vi "BNC555.ProcEvents.vi"(0 "i ref in":refnum<vi>, 5 "error in":errorcluster) -> (14 "i ref out":refnum<vi>, 19 "error out":errorcluster)   [LabVIEW 2014, in "BNC555.lvlib"]
doc: "This method is used to define the events the object will listen to. Add your own events here."
uses:
  BNC555.lvlib
  CS_Core/BaseProcess/BaseProcess.event definition.ctl
  CS_Core/CAEObj/CAEObj.event definition.ctl
  CS_Core/BaseProcess/BaseProcess.descriptor string definition.ctl
  CS_Core/BaseProcess/BaseProcess.lvlib
  CS_Core/CAEObj/CAEObj.lvlib
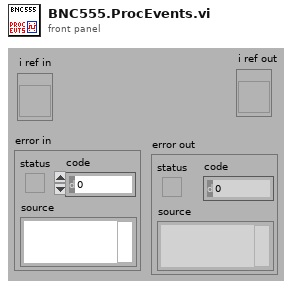
[diagram p1: front panel]
types:
  T1 = typedef "BaseProcess.lvlib/BaseProcess.event definition.ctl" = cluster{"CAEEvtDef":T2, "Data Descriptor":T3}
  T2 = typedef "CAEObj.lvlib/CAEObj.event definition.ctl" = cluster{"URL":string, "enable":bool, "ignoreResID":bool}
  T3 = typedef "BaseProcess.lvlib/BaseProcess.descriptor string definition.ctl" = string
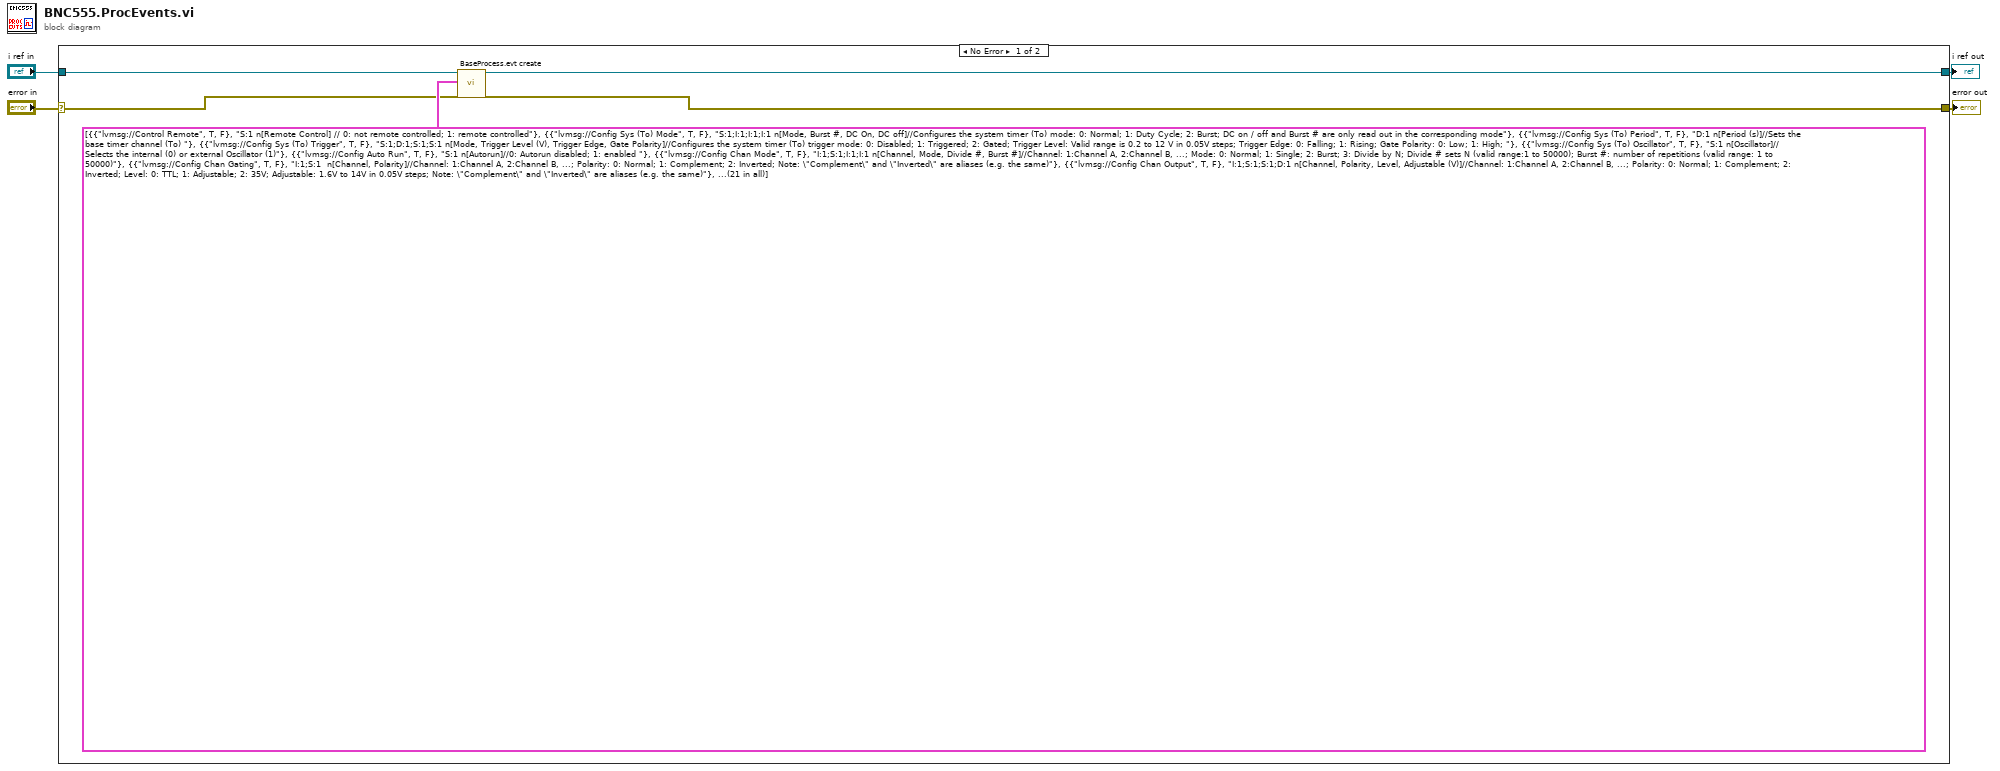
[diagram p0: block diagram]
diagram:
  n1 = case shown="No Error" "error in" {
    selector: "error in" -> [w5 w10]
    tunnel: "i ref in" -> [w9 w11]
    tunnel: [w8 w11] -> w3
    tunnel: [w7 w10] -> w2
    frame No Error {
      n2 = call "BaseProcess.evt create.vi"("i ref in"=w9, "newEvents"=T1[] [{"CAEEvtDef"={"URL"="lvmsg://Control Remote", "enable"=TRUE, "ignoreResID"=FALSE}, "Data Descriptor"="S:1 n[Remote Control] // 0: not remote controlled; 1: remote controlled"}, {"CAEEvtDef"={"URL"="lvmsg://Config Sys (To) Mode", "enable"=TRUE, "ignoreResID"=FALSE}, "Data Descriptor"="S:1;I:1;I:1;I:1 n[Mode, Burst #, DC On, DC off]//Configures the system timer (To) mode: 0: Normal; 1: Duty Cycle; 2: Burst; DC on / off and Burst # are only read out in the corresponding mode"}, {"CAEEvtDef"={"URL"="lvmsg://Config Sys (To) Period", "enable"=TRUE, "ignoreResID"=FALSE}, "Data Descriptor"="D:1 n[Period (s)]//Sets the base timer channel (To) "}, {"CAEEvtDef"={"URL"="lvmsg://Config Sys (To) Trigger", "enable"=TRUE, "ignoreResID"=FALSE}, "Data Descriptor"="S:1;D:1;S:1;S:1 n[Mode, Trigger Level (V), Trigger Edge, Gate Polarity]//Configures the system timer (To) trigger mode: 0: Disabled; 1: Triggered; 2: Gated; Trigger Level: Valid range is 0.2 to 12 V in 0.05V steps; Trigger Edge: 0: Falling; 1: Rising; Gate Polarity: 0: Low; 1: High; "}, {"CAEEvtDef"={"URL"="lvmsg://Config Sys (To) Oscillator", "enable"=TRUE, "ignoreResID"=FALSE}, "Data Descriptor"="S:1 n[Oscillator]//Selects the internal (0) or external Oscillator (1)"}, {"CAEEvtDef"={"URL"="lvmsg://Config Auto Run", "enable"=TRUE, "ignoreResID"=FALSE}, "Data Descriptor"="S:1 n[Autorun]//0: Autorun disabled; 1: enabled "}, {"CAEEvtDef"={"URL"="lvmsg://Config Chan Mode", "enable"=TRUE, "ignoreResID"=FALSE}, "Data Descriptor"="I:1;S:1;I:1;I:1 n[Channel, Mode, Divide #, Burst #]//Channel: 1:Channel A, 2:Channel B, ...; Mode: 0: Normal; 1: Single; 2: Burst; 3: Divide by N; Divide # sets N (valid range:1 to 50000); Burst #: number of repetitions (valid range: 1 to 50000)"}, {"CAEEvtDef"={"URL"="lvmsg://Config Chan Gating", "enable"=TRUE, "ignoreResID"=FALSE}, "Data Descriptor"="I:1;S:1  n[Channel, Polarity]//Channel: 1:Channel A, 2:Channel B, ...; Polarity: 0: Normal; 1: Complement; 2: Inverted; Note: \"Complement\" and \"Inverted\" are aliases (e.g. the same)"}, {"CAEEvtDef"={"URL"="lvmsg://Config Chan Output", "enable"=TRUE, "ignoreResID"=FALSE}, "Data Descriptor"="I:1;S:1;S:1;D:1 n[Channel, Polarity, Level, Adjustable (V)]//Channel: 1:Channel A, 2:Channel B, ...; Polarity: 0: Normal; 1: Complement; 2: Inverted; Level: 0: TTL; 1: Adjustable; 2: 35V; Adjustable: 1.6V to 14V in 0.05V steps; Note: \"Complement\" and \"Inverted\" are aliases (e.g. the same)"}, {"CAEEvtDef"={"URL"="lvmsg://Config Chan Pulse", "enable"=TRUE, "ignoreResID"=FALSE}, "Data Descriptor"="I:1;D:1;D:1 n[Channel, Delay (s), Width (s)]//Channel: 1:Channel A, 2:Channel B, ...; Valid range for Width and Delay: 4ns to 99,999999999 s"}, {"CAEEvtDef"={"URL"="lvmsg://Config Keypad and Display", "enable"=TRUE, "ignoreResID"=FALSE}, "Data Descriptor"="S:1;D:1;S:1;D:1 n[Key Beep, Beeper Volume, Key Lock, Display Intensity]//Configures display and keyboard attributes. 0: Key beep off, 1: on; "}, {"CAEEvtDef"={"URL"="lvmsg://Run or Stop", "enable"=TRUE, "ignoreResID"=FALSE}, "Data Descriptor"="S:1 n[Start/Stop]//Starts (1) or stops (2) the device "}, {"CAEEvtDef"={"URL"="lvmsg://Send SW Trigger", "enable"=TRUE, "ignoreResID"=FALSE}, "Data Descriptor"="//Sends a software trigger to the device"}, {"CAEEvtDef"={"URL"="lvmsg://Read Sys (To) Parameters", "enable"=TRUE, "ignoreResID"=FALSE}, "Data Descriptor"="//Reads the system parameters (To) and writes them to the GUI, update the DIM state and stores the information in own attributes."}, {"CAEEvtDef"={"URL"="lvmsg://Chan On or Off", "enable"=TRUE, "ignoreResID"=FALSE}, "Data Descriptor"="I:1;S:1 n[Channel, Activity]//Channel: 1:Channel A, 2:Channel B, ...; 0: Channel disabled, 1: enabled"}, {"CAEEvtDef"={"URL"="lvmsg://Chan Gating On or Off", "enable"=TRUE, "ignoreResID"=FALSE}, "Data Descriptor"="I:1;S:1 n[Channel, Gating Activity]//Channel: 1:Channel A, 2:Channel B, ...; 0: Channel Gating disabled, 1: enabled"}, {"CAEEvtDef"={"URL"="lvmsg://Read Chan Parameters", "enable"=TRUE, "ignoreResID"=FALSE}, "Data Descriptor"="//Reads the channel parameters of all channels, writes them to the GUI, updates the DIM services and stores the information in own attributes."}, {"CAEEvtDef"={"URL"="lvmsg://Read or Save Memory", "enable"=TRUE, "ignoreResID"=FALSE}, "Data Descriptor"="I:1;S:1 n[Memory, Activity]//Device internal memory location (1 to 10); 0: Read; 1: Save"}, {"CAEEvtDef"={"URL"="lvmsg://Self-Test", "enable"=TRUE, "ignoreResID"=FALSE}, "Data Descriptor"="//Forces the hardware to do a self-test and writes the result to the GUI"}, {"CAEEvtDef"={"URL"="lvmsg://Revision Query", "enable"=TRUE, "ignoreResID"=FALSE}, "Data Descriptor"="//Queries the hardware and firmware revision and device options and writes the information to the GUI"}, {"CAEEvtDef"={"URL"="lvmsg://Reset", "enable"=TRUE, "ignoreResID"=FALSE}, "Data Descriptor"="//Forces the hardware to do a reset"}] ("new events(V3.0)"), "error in (no error)"=w5) -> ("i ref out"=w8:refnum<vi>, "error out"=w7:errorcluster)  [unwired: 13 in, 2 out]
    }
    frame Error {
    }
  }
  "i ref out" <- w3
  "error out" <- w2
